vi "160-Outer Test.vi"(8 "error in":errorcluster) -> (0 "error out":errorcluster)   [LabVIEW 2020]
uses:
  classes/Test/Test.lvclass
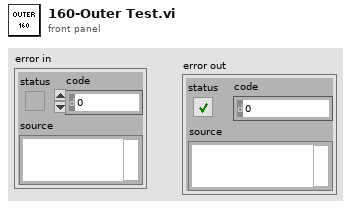
[diagram p1: front panel]
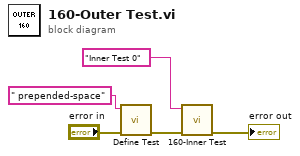
[diagram p0: block diagram]
diagram:
  n1 = call "Define Test.vi"("error in (no error)"="error in", "Label (VI Title)"=" prepended-space") -> ("error out"=w3:errorcluster)  [unwired: 8 in, 1 out]
  n2 = call "160-Inner Test.vi"("error in (no error)"=w3, "Label (VI Title)"="Inner Test 0") -> ("error out"=→"error out":errorcluster)  [unwired: 9 in]
